vi "reset buffer.vi"(8 "error in (no error)":errorcluster, 11 "DevRefnum":u64) -> (0 "error out":errorcluster, 3 "DevRefnum":u64)   [LabVIEW 2013, in "rtlsdr.lvlib"]
doc: "RTLSDR_API int rtlsdr_reset_buffer(rtlsdr_dev_t *dev);"
uses:
  <instrlib>/rtlsdr/rtlsdr.lvlib
  <instrlib>/rtlsdr/VIs/rtlsdr.dll
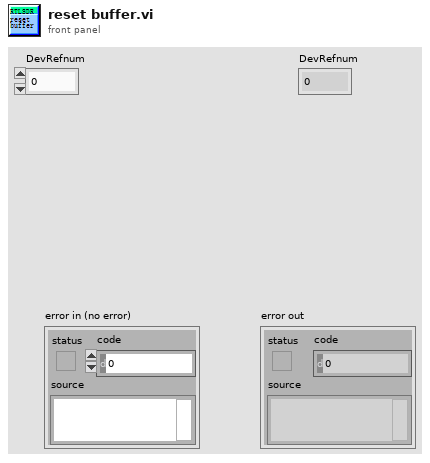
[diagram p1: front panel]
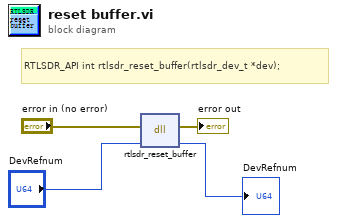
[diagram p0: block diagram]
diagram:
  # "RTLSDR_API int rtlsdr_reset_buffer(rtlsdr_dev_t *dev);"
  n1 = dll-call lib="C:/Program Files (x86)/National Instruments/LabVIEW 2013/instr.lib/rtlsdr/VIs/rtlsdr.*" fn="rtlsdr_reset_buffer"(error in="error in (no error)", "DevRefnum"="DevRefnum") -> (error out=→"error out":errorcluster, "DevRefnum"=→"DevRefnum":u64)  [unwired: 3 in, 1 out]
